vi "Untitled 4.vi"(0 "Lower_Intake_Man":bool, 1 "Raise_Intake_Man":bool, 3 "Flipper_Man":bool, 4 "Lower_Intake_Def":bool, 5 "Raise_Intake_Def":bool, 6 "Intake_Motor_Man":dbl, 7 "Stage_Motor_Man":dbl) -> (10 "Flipper_Man":enum16{"Closed", "Open"}(ring), 11 "Flipper_Man_Act":bool, 12 "Intake_Arm_Man":T3, 13 "Intake_Arm_Man_Act":bool, 14 "Intake_Def_Man":T2, 15 "Intake_Def_Man_Act":bool, 16 "Intake_Motor_Man_Act":bool, 17 "Stage_Motor_Man_Act":bool, 18 "Stage_Motor_Man":T1, 19 "Intake_Motor_Man":T1)   [LabVIEW 2015]
uses:
  Intake Enum..ctl
  Arm_defense_Type_Def.ctl
  Motor_Dir_Type_Def.ctl
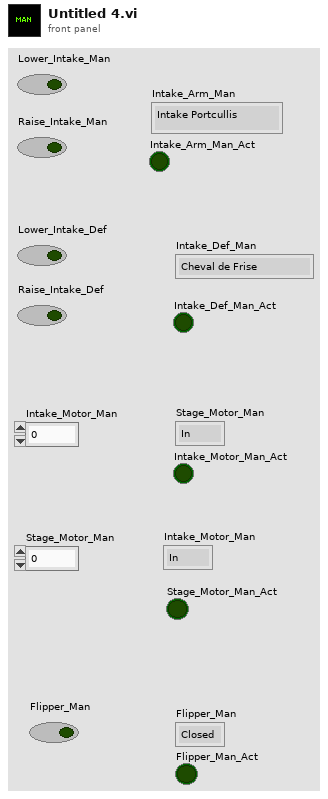
[diagram p1: front panel]
types:
  T1 = typedef "Motor_Dir_Type_Def.ctl" = enum16{"In", "Out", "Off"}
  T2 = typedef "Arm_defense_Type_Def.ctl" = enum16{"Cheval de Frise", "Portcullis", "Ball_Pickup"}
  T3 = typedef "Intake Enum..ctl" = enum16{"Intake Portcullis", "Intake Ball Pickup", "Intake Cheval", " Intake Raised"}
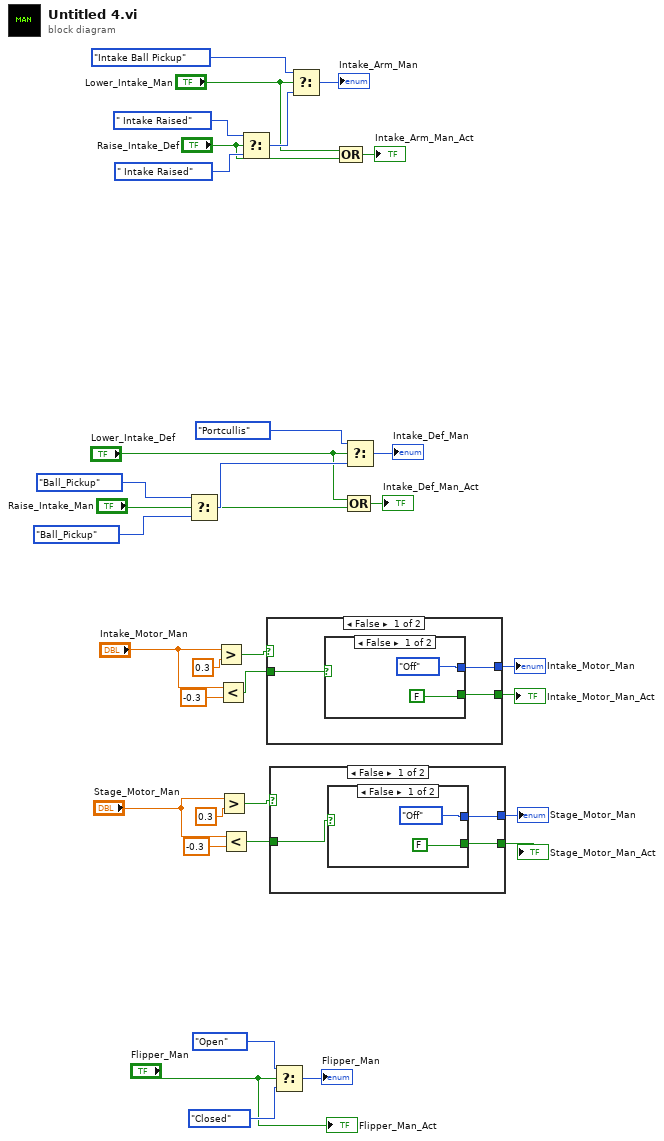
[diagram p0: block diagram]
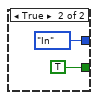
[diagram p2: hidden frame]
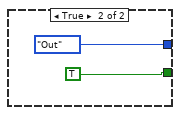
[diagram p3: hidden frame]
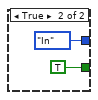
[diagram p4: hidden frame]
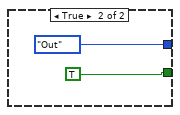
[diagram p5: hidden frame]
diagram:
  n1 = Select(t=Arm_defense_Type_Def."Ball_Pickup" ("P1_Value"), s="Raise_Intake_Man", f=Arm_defense_Type_Def."Ball_Pickup" ("P1_Value")) -> (s? t:f=w27:T2)
  n2 = Greater?(x="Intake_Motor_Man", y=0.3 ("x")) -> (0:w21:bool)
  n3 = Less?(x="Intake_Motor_Man", y=-0.3) -> (x < y?=w6:bool)
  n4 = Greater?(x="Stage_Motor_Man", y=0.3 ("x")) -> (0:w20:bool)
  n5 = Less?(x="Stage_Motor_Man", y=-0.3) -> (x < y?=w5:bool)
  n6 = Select(t=Intake_Enum.." Intake Raised" ("P1_Value"), s="Raise_Intake_Def", f=Intake_Enum.." Intake Raised" ("P1_Value")) -> (s? t:f=w34:T3)
  n7 = case shown="False" w21 {
    tunnel: [w37 Motor_Dir_Type_Def."Out" ("P1_Value")] -> w16
    tunnel: [w36 TRUE] -> w15
    tunnel: w6 -> [w35 _]
    frame False {
      n8 = case shown="False" w35 {
        tunnel: [Motor_Dir_Type_Def."Off" ("P1_Value") Motor_Dir_Type_Def."In" ("P1_Value")] -> w37
        tunnel: [FALSE TRUE] -> w36
        frame False {
        }
        frame True {
        }
      }
    }
    frame True {
    }
  }
  "Intake_Motor_Man" <- w16
  "Intake_Motor_Man_Act" <- w15
  n9 = case shown="False" w20 {
    tunnel: [w46 Motor_Dir_Type_Def."Out" ("P1_Value")] -> w14
    tunnel: [w45 TRUE] -> w13
    tunnel: w5 -> [w44 _]
    frame False {
      n10 = case shown="False" w44 {
        tunnel: [Motor_Dir_Type_Def."Off" ("P1_Value") Motor_Dir_Type_Def."In" ("P1_Value")] -> w46
        tunnel: [FALSE TRUE] -> w45
        frame False {
        }
        frame True {
        }
      }
    }
    frame True {
    }
  }
  "Stage_Motor_Man" <- w14
  "Stage_Motor_Man_Act" <- w13
  n11 = Select(t=enum16{"Closed", "Open"}."Open" ("P1_Value"), s="Flipper_Man", f=enum16{"Closed", "Open"}."Closed" ("P1_Value")) -> (s? t:f=→"Flipper_Man":enum16{"Closed", "Open"})
  n12 = Select(t=Intake_Enum.."Intake Ball Pickup" ("P1_Value"), s="Lower_Intake_Man", f=w34) -> (s? t:f=→"Intake_Arm_Man":T3)
  n13 = Compound Arithmetic op=OR("Lower_Intake_Man", "Raise_Intake_Def") -> (→"Intake_Arm_Man_Act":bool)
  n14 = Select(t=Arm_defense_Type_Def."Portcullis" ("P1_Value"), s="Lower_Intake_Def", f=w27) -> (s? t:f=→"Intake_Def_Man":T2)
  n15 = Compound Arithmetic op=OR("Lower_Intake_Def", "Raise_Intake_Man") -> (→"Intake_Def_Man_Act":bool)
  "Flipper_Man_Act" <- "Flipper_Man"
